vi "BaseTemplate_GetObjectStatus.vi"(0 "reference in":refnum<class "BaseTemplate.lvclass">, 2 "Simple Info":bool, 5 "error in (no error)":errorcluster) -> (9 "Nr of users":i32, 10 "All objects names":string[](array[string]), 11 "One user":bool, 12 "# of objects":i32, 13 "Class name":string, 14 "reference out":refnum<class "BaseTemplate.lvclass">, 15 "Not a refnum?":bool, 16 "Object name":string, 17 "All refs out":refnum<class "BaseTemplate.lvclass">[](array[class]), 18 "Attributes locked?":bool, 19 "error out":errorcluster)   [LabVIEW 2020, in "BaseTemplate.lvclass"]
doc: "Returns the object status and also information about all the objects in the class."
uses:
  <resource>/Framework/Providers/Open_GDS/ClassProviders/Provider_EndevoGOOP300/Templates/BaseTemplate/BaseTemplate.lvclass
  <vilib>/addons/_goop3.llb/3GOOPStates.ctl
  <resource>/Framework/Providers/Open_GDS/ClassProviders/Provider_EndevoGOOP300/Templates/BaseTemplate/BaseTemplate.lvclass/BaseTemplate.ctl
panel:
  in  "DebuggerInput":string
  out "DebuggerOutput":string
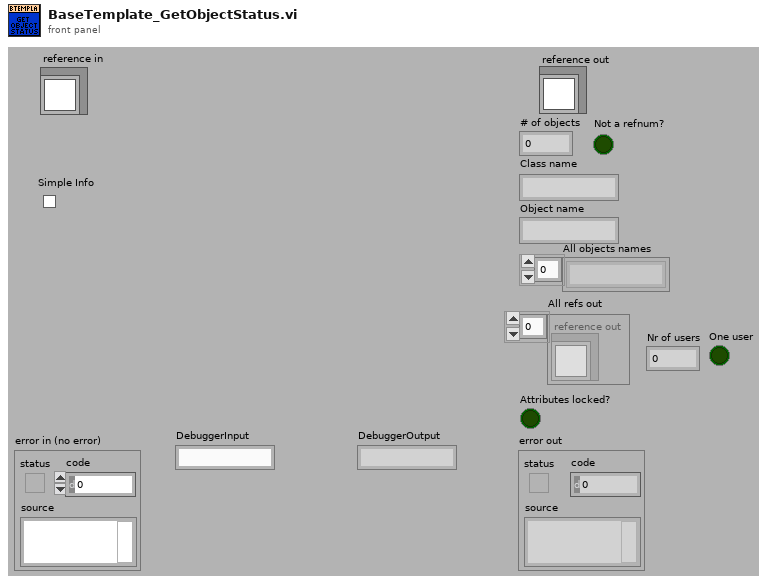
[diagram p1: front panel]
types:
  T1 = typedef "3GOOPStates.ctl" = enum16{"Set", "Get", "New", "Delete", "Clear", "Test and get", "Unlock data", "Information", "Look up existing", "New or look up existing", "Test and get shared", "Get shared", "Set shared", "Unlock shared", "Find dynamic method", "Register dynamic method", "Preload dynamic method", "Probe", "Cast to more generic", "Cast to more specific"}
  T2 = cluster{"Mode":enum16{"Get", "Set", "Delete"}, "Ref":i32, "ObjAttribute":string, "ClassAttribute":string}
  T3 = cluster{"Object names":string[], "Refs":i32[], "ObjectAttributeLocked":bool, "ClassAttributeLocked":bool, "ObjAttribute":variant, "ClassAttribute":variant}
  T4 = typedef "3GOOPClassStatistics.ctl" = cluster{"# of waiting":u32, "Object names":string[], "Base class folders":path[], "Refs":i32[], "Class name":string}
  T5 = typedef "BaseTemplate.lvclass/ObjectAttributes.ctl" = cluster{"Attribute1":dbl}
  T6 = typedef "BaseTemplate.lvclass/ClassAttributes.ctl" = cluster{"classAttribute1":bool}
  T7 = typedef "BaseTemplate.lvclass/ObjectReference.ctl" = refnum<k1>
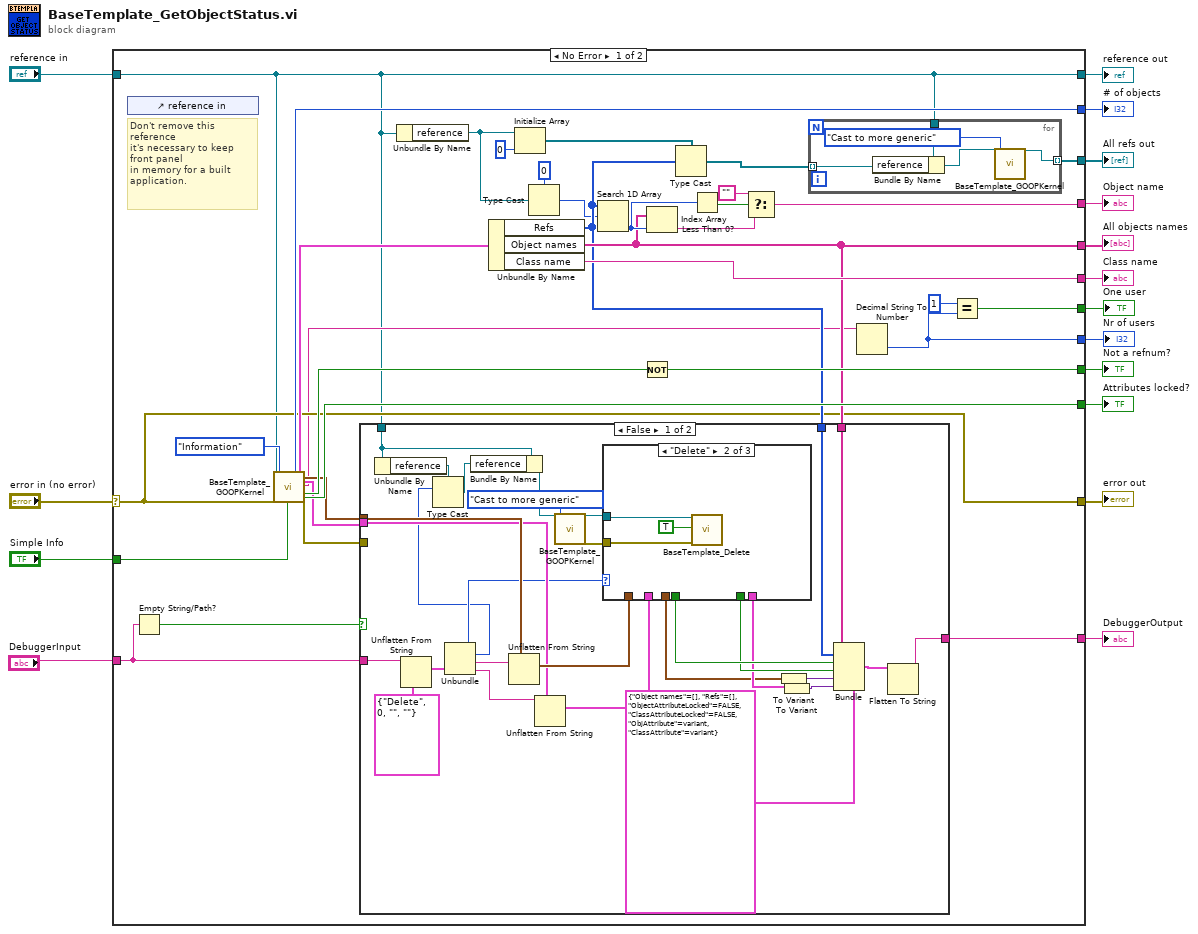
[diagram p0: block diagram]
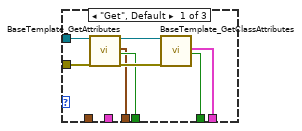
[diagram p2: hidden frame]
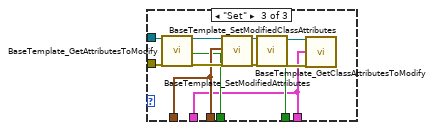
[diagram p3: hidden frame]
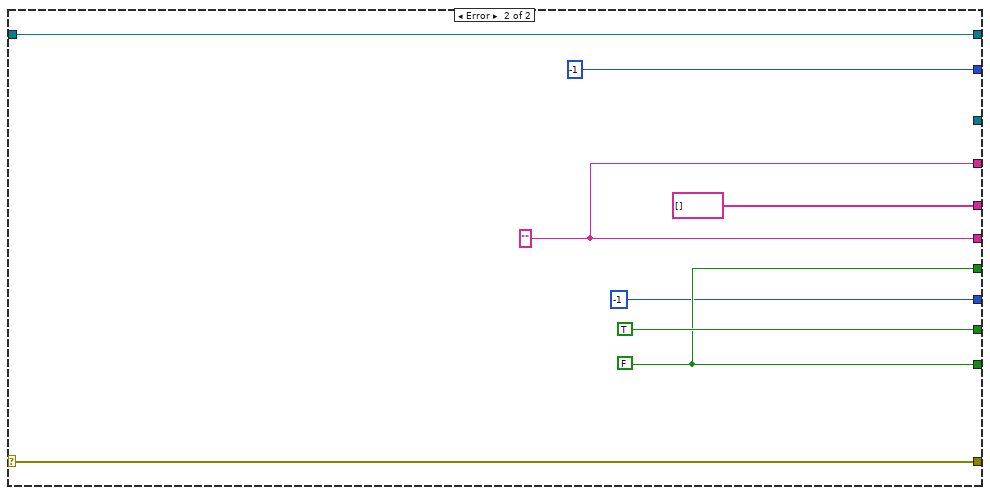
[diagram p5: hidden frame]
diagram:
  n1 = case shown="No Error" "error in (no error)" {
    selector: "error in (no error)" -> [w26 w115]
    tunnel: [w26 w115] -> w15
    tunnel: "reference in" -> [w18 w113]
    tunnel: [w18 w113] -> w13
    tunnel: [w49 -1 ("# of objects")] -> w12
    tunnel: [w45 TRUE ("Exists?")] -> w11
    tunnel: [w46 w109] -> w10
    tunnel: [w44 w110] -> w9
    tunnel: [w31 string[] [] ("Object names")] -> w8
    tunnel: [w27 _] -> w7
    tunnel: [w39 w110] -> w6
    tunnel: "DebuggerInput" -> [w36 _]
    tunnel: [w29 _] -> w4
    tunnel: [w24 -1] -> w3
    tunnel: [w23 w109] -> w2
    tunnel: "Simple Info" -> [w17 _]
    frame No Error {
      # "Don't remove this reference\nit's necessary to keep front panel\nin memory for a built application."
      n2 = control-ref of="reference in"() -> ()  [unwired: 1 out]
      n3 = Empty String/Path?(string/path=w36) -> (empty?=w35:bool)
      n4 = call <resource>:"BaseTemplate_GOOPKernel.vi"("Ref in"=w18, "error in (no error)"=w26, "Action"=3GOOPStates."Information", "Misc"=w17) -> ("# of objects"=w49:i32, "Class statistics"=w47:T4, "Data out"=w34:T5, "Data shared out"=w33:T6, "Probe out"=w25:string, "Exists?"=w48:bool, "Data locked?"=w46:bool, "error out"=w32:errorcluster)  [unwired: 13 in, 3 out]
      n5 = Unbundle By Name(w18) -> ("reference"=w19:T7)
      n6 = Unbundle By Name(w47) -> ("Refs"=w30:i32[], "Object names"=w31:string[], "Class name"=w44:string)
      n7 = case shown="False" w35 {
        tunnel: w32 -> [_ _]
        tunnel: w18 -> [w61 _]
        tunnel: [w80 _] -> w29
        tunnel: w34 -> [w75 _]
        tunnel: w33 -> [w74 _]
        tunnel: w36 -> [w72 _]
        tunnel: w30 -> [w70 _]
        tunnel: w31 -> [w69 _]
        frame False {
          n8 = Unbundle By Name(w61) -> ("reference"=w60:T7)
          n9 = Unflatten From String(type=T2 {"Mode"=enum."Delete", "Ref"=0, "ObjAttribute"="", "ClassAttribute"=""} ("DebuggerIn"), binary string=w72) -> (value=w77:T2)  [unwired: 3 in, 2 out]
          n10 = Unbundle(w77) -> ("Mode"=w73:enum16{"Get", "Set", "Delete"}, "Ref"=w62:i32, "ObjAttribute"=w78:string, "ClassAttribute"=w79:string)
          n11 = Type Cast(type=w60, x=w62) -> (*(type *) &x=w63:T7)
          n12 = Bundle By Name(cluster=w61, "reference"=w63) -> (w59:refnum<class "BaseTemplate.lvclass">)
          n13 = Unflatten From String(type=w75, binary string=w78) -> (value=w76:T5)  [unwired: 3 in, 2 out]
          n14 = Unflatten From String(type=w74, binary string=w79) -> (value=w71:T6)  [unwired: 3 in, 2 out]
          n15 = call <resource>:"BaseTemplate_GOOPKernel.vi"("Ref in"=w59, "Action"=3GOOPStates."Cast to more generic") -> ("Ref out"=w56:refnum<class "BaseTemplate.lvclass">, "error out"=w57:errorcluster)  [unwired: 15 in, 9 out]
          n16 = case shown="\"Delete\"" w73 {
            tunnel: w57 -> [w92 w94 w106]
            tunnel: w56 -> [w91 w95 w107]
            tunnel: [w88 _ w98] -> w82
            tunnel: [w87 _ w97] -> w81
            tunnel: [w86 _ w99] -> w65
            tunnel: [w85 _ w96] -> w68
            tunnel: w76 -> [_ _ w99]
            tunnel: w71 -> [_ _ w96]
            frame "Get", Default {
              n17 = call <resource>:"BaseTemplate_GetAttributes.vi"("reference in"=w91, "error in (no error)"=w92) -> ("reference out"=w90:refnum<class "BaseTemplate.lvclass">, "Attributes"=w86:T5, "Attributes locked?"=w88:bool, "error out"=w89:errorcluster)  [unwired: 14 in]
              n18 = call <resource>:"BaseTemplate_GetClassAttributes.vi"("reference in"=w90, "error in (no error)"=w89) -> ("Class attributes"=w85:T6, "Attributes locked?"=w87:bool)  [unwired: 14 in, 2 out]
            }
            frame "Delete" {
              n19 = call <resource>:"BaseTemplate_Delete.vi"("reference in"=w95, "Force delete"=TRUE, "error in (no error)"=w94) -> ()  [unwired: 14 in, 3 out]
            }
            frame "Set" {
              n20 = call <resource>:"BaseTemplate_GetAttributesToModify.vi"("reference in"=w107, "error in (no error)"=w106) -> ("reference out"=w105:refnum<class "BaseTemplate.lvclass">, "Timeout"=w98:bool, "error out"=w104:errorcluster)  [unwired: 14 in, 1 out]
              n21 = call <resource>:"BaseTemplate_SetModifiedAttributes.vi"("reference in"=w105, "Attributes"=w99, "error in (no error)"=w104) -> ("reference out"=w103:refnum<class "BaseTemplate.lvclass">, "error out"=w102:errorcluster)  [unwired: 15 in]
              n22 = call <resource>:"BaseTemplate_GetClassAttributesToModify.vi"("reference in"=w103, "error in (no error)"=w102) -> ("reference out"=w101:refnum<class "BaseTemplate.lvclass">, "Timeout"=w97:bool, "error out"=w100:errorcluster)  [unwired: 14 in, 1 out]
              n23 = call <resource>:"BaseTemplate_SetModifiedClassAttributes.vi"("reference in"=w101, "Class attributes"=w96, "error in (no error)"=w100) -> ()  [unwired: 15 in, 2 out]
            }
          }
          n24 = To Variant(anything=w65) -> (Variant=w66:variant)
          n25 = To Variant(anything=w68) -> (Variant=w67:variant)
          n26 = Bundle(cluster=T3 {"Object names"=[], "Refs"=[], "ObjectAttributeLocked"=FALSE, "ClassAttributeLocked"=FALSE, "ObjAttribute"=variant, "ClassAttribute"=variant}, "Object names"=w69, "Refs"=w70, "ObjectAttributeLocked"=w82, "ClassAttributeLocked"=w81, "ObjAttribute"=w66, "ClassAttribute"=w67) -> (w84:T3)
          n27 = Flatten To String(anything=w84) -> (data string=w80:string)  [unwired: 3 in, 2 out]
        }
        frame True {
        }
      }
      n28 = Initialize Array(w19, 0 ("Dimension Size")) -> (w37:T7[])
      n29 = Type Cast(type=0, x=w19) -> (*(type *) &x=w20:i32)
      n30 = Search 1D Array(1D array=w30, element=w20) -> (index of element=w43:i32)  [unwired: 1 in]
      n31 = Not(x=w48) -> (.not. x?=w45:bool)
      n32 = Index Array(array=w31, index=w43) -> (element=w41:string)
      n33 = Type Cast(type=w37, x=w30) -> (*(type *) &x=w28:T7[])
      n34 = Less Than 0?(x=w43) -> (x < 0?=w42:bool)
      n35 = Select(t="", s=w42, f=w41) -> (s? t:f=w39:string)
      n36 = for {
        tunnel: w28 -> [w55] mode=indexing
        tunnel: [w53] -> w27 mode=indexing
        tunnel: w18 -> [w51]
        n37 = Bundle By Name(cluster=w51, "reference"=w55) -> (w54:refnum<class "BaseTemplate.lvclass">)
        n38 = call <resource>:"BaseTemplate_GOOPKernel.vi"("Ref in"=w54, "Action"=3GOOPStates."Cast to more generic") -> ("Ref out"=w53:refnum<class "BaseTemplate.lvclass">)  [unwired: 15 in, 10 out]
      }
      n39 = Decimal String To Number(string=w25) -> (number=w24:i32)  [unwired: 2 in, 1 out]
      n40 = Equal?(x=1, y=w24) -> (x = y?=w23:bool)
    }
    frame Error {
      w110 = "" ("Class name")
      w109 = FALSE
    }
  }
  "error out" <- w15
  "reference out" <- w13
  "# of objects" <- w12
  "Not a refnum?" <- w11
  "All refs out" <- w7
  "Attributes locked?" <- w10
  "Class name" <- w9
  "All objects names" <- w8
  "Object name" <- w6
  "DebuggerOutput" <- w4
  "One user" <- w2
  "Nr of users" <- w3
